vi "Sym2fft2.vi"(0 "Parallel Symbol In":cdb[](array[numeric]), 1 "D/A Rate":dbl format="%#_13g", 2 "Carrier Symbol":cdb format="%#_13g", 3 "Fundamental Frequency":dbl format="%#_13g", 4 "Number of Subcarriers":i32) -> (5 "Time Domain Out":cdb[](array[numeric]), 6 "DC Offset":cdb format="%#_13g")   [LabVIEW 2013]
uses:
  <vilib>/Analysis/2dsp.llb/Inverse Complex FFT.vi
  <vilib>/Analysis/NI_AALPro.lvlib
panel:
  in  "shift?":bool
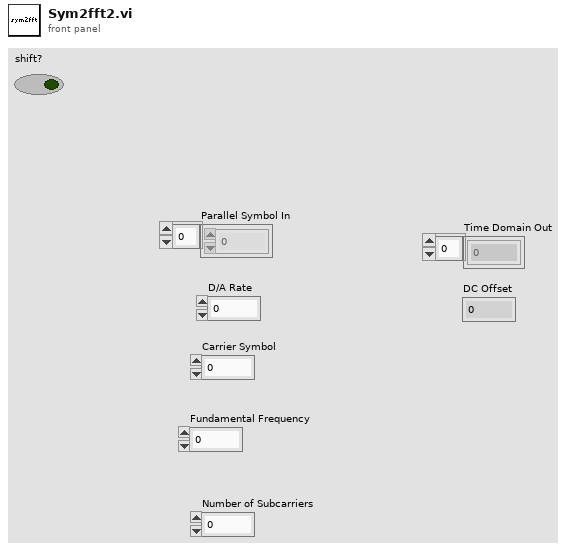
[diagram p1: front panel]
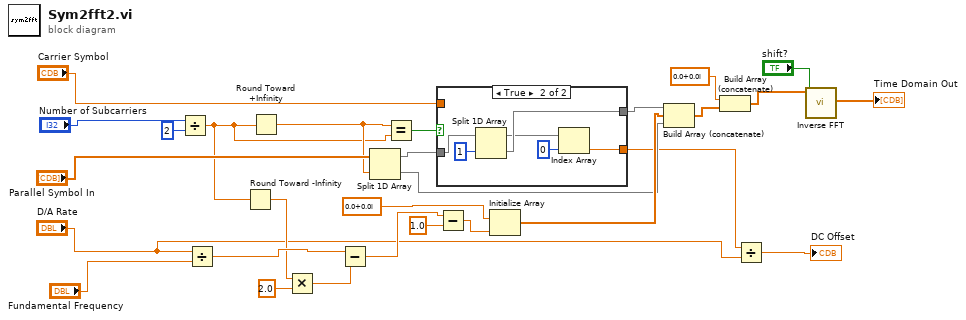
[diagram p0: block diagram]
diagram:
  n1 = Divide(x="Number of Subcarriers", y=2) -> (x/y=w17:dbl)
  n2 = Divide(x="D/A Rate", y="Fundamental Frequency") -> (x/y=w27:dbl)
  n3 = Round Toward -Infinity(1:w17) -> (0:w23:dbl)
  n4 = Round Toward +Infinity(x=w17) -> (ceil(x): smallest int >= x=w18:dbl)
  n5 = Multiply(x=w23, y=2.0) -> (x*y=w28:dbl)
  n6 = Subtract(x=w27, y=w28) -> (x-y=w21:dbl)
  n7 = Split 1D Array(array="Parallel Symbol In", index=w18) -> (first subarray=w14:cdb[], second subarray=w10:cdb[])
  n8 = Equal?(x=w18, y=w17) -> (x = y?=w2:bool)
  n9 = case shown="True" w2 {
    tunnel: w14 -> [w30 w34]
    tunnel: "Carrier Symbol" -> [w29 _]
    tunnel: [w30 w33] -> w12
    tunnel: [w29 w31] -> w7
    frame False {
    }
    frame True {
      n10 = Split 1D Array(array=w34, index=1) -> (first subarray=w32:cdb[], second subarray=w33:cdb[])
      n11 = Index Array(array=w32, index=0) -> (element=w31:cdb)
    }
  }
  n12 = Subtract(x=w21, y=1.0) -> (x-y=w16:dbl)
  n13 = Initialize Array(cdb 0.0+0.0i ("Carrier Symbol 2"), w16) -> (w11:cdb[])
  n14 = Build Array (concatenate)(w12, w11, w10) -> (w3:cdb[])
  n15 = Build Array (concatenate)(cdb 0.0+0.0i ("Carrier Symbol 2"), w3) -> (w4:cdb[])
  n16 = Divide(x=w7, y="D/A Rate") -> (x/y=→"DC Offset":cdb)
  n17 = call-poly <vilib>:"Inverse FFT.vi"("shift?"="shift?", "FFT {X}"=w4) -> ("X"=→"Time Domain Out":cdb[])  [unwired: 8 in, 1 out]
